vi "Module_ENG_TCPClient.vi"(8 "error in (no error)":errorcluster, 9 "Module ID (-1: Do not Address)":i32=-1, 10 "Wait on Module(s) (\"\": none)":string, 11 "Auto Reconnect?":bool) -> (0 "error out":errorcluster)   [LabVIEW 2019, in "Module_ENG_TCPClient.lvclass"]
doc: "created using\nJSMA Module Template - ENGINE Class 0.2.1.12\nRob Humfeld - Jet Engineering\nCopyright (c) 2020, Jet Engineering"
uses:
  Module_ENG_TCPClient.lvclass
  <userlib>/Jet Engineering/JSMA/Libraries/jModule Class/Typedefs/jModule_TimerConfig STYP.ctl
  <userlib>/Jet Engineering/JSMA/Libraries/jModule Class/Typedefs/jModule_TimerType STYP.ctl
  Private/Module_ENG_TCPClient_jMsgTxList STYP.ctl
  <userlib>/Jet Engineering/JSMA/Libraries/jMsg_CORE/jMsg_JSMA_ModuleOnline/jMsg_JSMA_ModuleOnline.lvclass
  Shared/jMsgs/jMsg_TCPConnection_Status/jMsg_TCPConnection_Status.lvclass
  C:/Program Files/National Instruments/LabVIEW 2019/user.lib/Jet Engineering/JSMA/Libraries/jMsg Class/jMsg.lvclass
  Shared/jMsgs/jMsg_TCPClient_Message_Receive/jMsg_TCPClient_Message_Receive.lvclass
  Private/Module_ENG_TCPClient_jMsgRxList STYP.ctl
  <userlib>/Jet Engineering/JSMA/Libraries/jMsg_CORE/jMsg_JSMA_ApplicationShutdown/jMsg_JSMA_ApplicationShutdown.lvclass
  Shared/jMsgs/jMsg_TCPClient_Message_Send/jMsg_TCPClient_Message_Send.lvclass
  Shared/jMsgs/jMsg_TCPClient_Connection_Update/jMsg_TCPClient_Connection_Update.lvclass
  C:/Program Files/National Instruments/LabVIEW 2019/user.lib/Jet Engineering/JSMA/Libraries/jModule Class/jModule.lvclass
  Private/Module_ENG_TCPClient_LocalData STYP.ctl
  Private/Module_ENG_TCPClient_EngineStatus STYP.ctl
  Shared/TCPConnectionSettings STYP.ctl
  Shared/TCPReceiver/TCPReceiver.lvclass
  <userlib>/Jet Engineering/JET_QSM/Code/Private/JET_QSM_InvalidOption STYP.ctl
  <userlib>/Jet Engineering/JSMA/Libraries/jModule Class/jModule.lvclass/jModule.ctl
  Module_ENG_TCPClient.lvclass/Module_ENG_TCPClient.ctl
  Shared/jMsgs/jMsg_TCPClient_Message_Send/jMsg_TCPClient_Message_Send.lvclass/jMsg_TCPClient_Message_Send.ctl
  Shared/jMsgs/jMsg_TCPClient_Connection_Update/jMsg_TCPClient_Connection_Update.lvclass/jMsg_TCPClient_Connection_Update.ctl
  <userlib>/Jet Engineering/JSMA/Libraries/jMsg Class/jMsg.lvclass/jMsg.ctl
  Shared/jMsgs/jMsg_TCPConnection_Status/jMsg_TCPConnection_Status.lvclass/jMsg_TCPConnection_Status.ctl
  <userlib>/Jet Engineering/JSMA/Libraries/jMsg_CORE/jMsg_JSMA_Exception/jMsg_JSMA_Exception.lvclass/jMsg_JSMA_Exception.ctl
  <userlib>/Jet Engineering/JSMA/Libraries/jMsg_CORE/jMsg_JSMA_SubscriptionChange/jMsg_JSMA_SubscriptionChange.lvclass/jMsg_JSMA_SubscriptionChange.ctl
  <userlib>/Jet Engineering/JSMA/Libraries/jMsg_CORE/jMsg_Addressed/jMsg_Addressed.lvclass/jMsg_Addressed.ctl
  Shared/TCPPacket/TCPPacket.lvclass
  Shared/jMsgs/jMsg_TCPClient_Message_Receive/jMsg_TCPClient_Message_Receive.lvclass/jMsg_TCPClient_Message_Receive.ctl
  <userlib>/Jet Engineering/JET_QSM/Code/Private/JET_QSM - Add State [String API].vi
  <userlib>/Jet Engineering/JSMA/Libraries/jModule Class/Read Timeout Configuration.vi
  <userlib>/Jet Engineering/JET_QSM/Code/Private/JET_QSM - Add State to Front [String API].vi
  <userlib>/Jet Engineering/JSMA/Libraries/jModule Class/Read jMsgRx.vi
  <userlib>/Jet Engineering/JSMA/Libraries/jMsg Class/(create) jMsg.vi
  <userlib>/Jet Engineering/JSMA/Libraries/jMsg_CORE/jMsg_JSMA_Exception/(create) jMsg_JSMA_Exception.vi
  <userlib>/Jet Engineering/JSMA/Libraries/jModule Class/jModule - Stats_Exception Count Increment.vi
  <userlib>/Jet Engineering/JSMA/Libraries/jModule Class/jModule - SimpleTx.vi
  <userlib>/Jet Engineering/JSMA/Libraries/jModule Class/jModule - Exception Enqueue.vi
  <userlib>/Jet Engineering/JSMA/Libraries/jMsg Class/Read No Listener Action.vi
  <userlib>/Jet Engineering/JSMA/Libraries/jModule Class/jModule - ExceptionBatchTx.vi
  <userlib>/Jet Engineering/JSMA/Libraries/jModule Class/jModule - Send to List.vi
  <userlib>/Jet Engineering/JSMA/Libraries/jModule Class/jModule - AddressedTx.vi
  <userlib>/Jet Engineering/JSMA/Libraries/jModule Class/jModule - Stats_Tx Count Increment.vi
  <userlib>/Jet Engineering/JSMA/Libraries/jMsg Class/Read Type.vi
  <userlib>/Jet Engineering/JSMA/Libraries/jMsg Class/Write SendID.vi
  <userlib>/Jet Engineering/JSMA/Libraries/jMsg Class/Read Name.vi
  <userlib>/Jet Engineering/JSMA/Libraries/jMasterTable_Subscription/jMasterTable_Subscription - Get Queue Type.vi
  <userlib>/Jet Engineering/JSMA/Libraries/jMsg Class/jMsg - Set Source.vi
  <userlib>/Jet Engineering/JSMA/Libraries/Shared/JSMA_GetClassName.vi
  <userlib>/Jet Engineering/JSMA/Libraries/jMsg Class/Read Sent Time.vi
  <userlib>/Jet Engineering/JSMA/Libraries/jMsg Class/Read Source.vi
  <userlib>/Jet Engineering/JSMA/Libraries/jMasterTable_Subscription/jMasterTable_Subscription - Remove Module.vi
  <userlib>/Jet Engineering/JSMA/Libraries/jMsg Class/Write Source.vi
  <userlib>/Jet Engineering/JSMA/Libraries/jMsg_CORE/jMsg_JSMA_SubscriptionChange/(create) jMsg_JSMA_SubscriptionChange.vi
  <userlib>/Jet Engineering/JSMA/Libraries/jMasterTable_Subscription/jMasterTable_Subscription - Get Sub List.vi
  <userlib>/Jet Engineering/JSMA/Libraries/jMsg_CORE/jMsg_Addressed/Read Qualified Name.vi
  <userlib>/Jet Engineering/JSMA/Libraries/jMsg_CORE/jMsg_Addressed/Read RecvID.vi
  <userlib>/Jet Engineering/JSMA/Libraries/jMasterTable_Subscription/jMasterTable_Subscription - Get-Create Queue.vi
  <userlib>/Jet Engineering/JSMA/Libraries/jMasterTable_Message/jMasterTable_Message - Add jMsg.vi
  <userlib>/Jet Engineering/JSMA/Libraries/jMasterTable_Message/jMasterTable_Message - Get-Create Queue.vi
  <userlib>/Jet Engineering/JSMA/Libraries/jMsg_CORE/jMsg_JSMA_Exception/jMsg_JSMA_Exception.lvclass
  <userlib>/Jet Engineering/JSMA/Libraries/jMsg_CORE/jMsg_JSMA_SubscriptionChange/jMsg_JSMA_SubscriptionChange.lvclass
  <userlib>/Jet Engineering/JSMA/Libraries/jMsg_CORE/jMsg_Addressed/jMsg_Addressed.lvclass
  <vilib>/Utility/error.llb/Trim Whitespace.vi
  <vilib>/Utility/error.llb/Error Cluster From Error Code.vi
  <vilib>/Utility/LVClass/Get LV Class Path.vi
  <userlib>/Jet Engineering/JSMA/Libraries/jSubscription Class/jSubscription.lvclass
  <userlib>/Jet Engineering/JSMA/Libraries/jModule Class/jModule.lvclass
  <userlib>/Jet Engineering/JSMA/Libraries/jMsg Class/jMsg.lvclass
panel:
  out "Timer Configuration":T1 {"Expiration Time" format="%<%.3X>T"}
  out "jModule Name":string
  out "iter":i32
  out "Latency, sec.":dbl
  out "RxTime":timestamp format="%<%H:%M:%S%3u>T"
  out "Last Rx Message":string
  out "Recent states before Error (with tick counts)":string
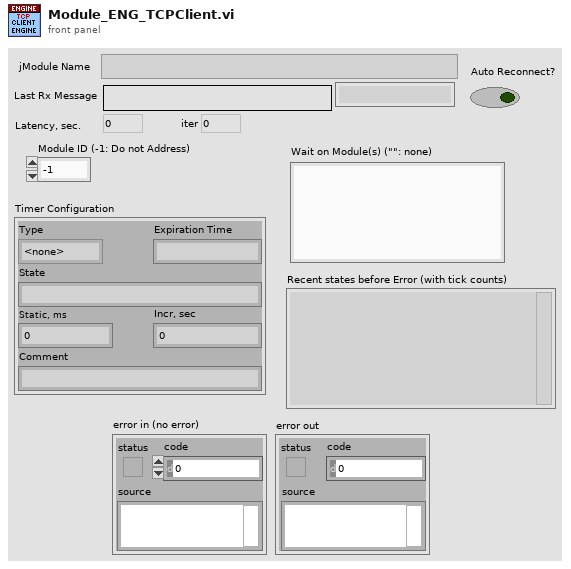
[diagram p1: front panel]
types:
  T1 = typedef "JSMA API.lvlib/jModule.lvclass/jModule_TimerConfig STYP.ctl" = cluster{"Type":T2, "Expiration Time":timestamp, "State":string, "Static, ms":i32, "Incr, sec":dbl, "Comment":string}
  T2 = typedef "JSMA API.lvlib/jModule.lvclass/jModule_TimerType STYP.ctl" = enum16{"<none>", "Static", "Countdown", "Periodic"}
  T3 = typedef "JET_QSM_InvalidOption STYP.ctl" = enum16{"Ignore", "Dialog", "Error"}
  T4 = typedef "Module_ENG_TCPClient.lvclass/Module_ENG_TCPClient_LocalData STYP.ctl" = cluster{"VI":cluster{"error":errorcluster, "isExiting?":bool}, "EngineStatus":T5}
  T5 = typedef "Module_ENG_TCPClient.lvclass/Module_ENG_TCPClient_EngineStatus STYP.ctl" = cluster{"Connection":T6, "Valid Settings?":bool, "Receiver":refnum<class "TCPReceiver.lvclass">}
  T6 = typedef "TCPConnectionSettings STYP.ctl" = cluster{"IP":string, "Port":u16, "Connection":refnum<k5>, "Connected?":bool}
  T7 = typedef "Module_ENG_TCPClient.lvclass/Module_ENG_TCPClient_jMsgRxList STYP.ctl" = cluster{"<placeholder>":refnum<class "jMsg_JSMA_ApplicationShutdown.lvclass">, "jMsg_TCPClient_Message_Send":refnum<class "jMsg_TCPClient_Message_Send.lvclass">, "jMsg_TCPClient_Connection_Update":refnum<class "jMsg_TCPClient_Connection_Update.lvclass">}
  T8 = typedef "Module_ENG_TCPClient.lvclass/Module_ENG_TCPClient_jMsgTxList STYP.ctl" = cluster{"<placeholder>":refnum<class "jMsg_JSMA_ModuleOnline.lvclass">, "jMsg_TCPConnection_Status":refnum<class "jMsg_TCPConnection_Status.lvclass">, "jMsg_TCPClient_Message_Receive":refnum<class "jMsg_TCPClient_Message_Receive.lvclass">}
  T9 = typedef "JET_QSM_Refnum STYP.ctl" = cluster{"state":cluster{"queue":refnum<queue>, "idle":string, "error":string, "STOP":string}, "debug":cluster{"enabled?":bool, "queue":refnum<queue>}, "Invalid.option":T3, "QSM.Name":string}
  T10 = typedef "JET_QSM_Element STYP.ctl" = cluster{"state":string, "data":variant, "comment":string}
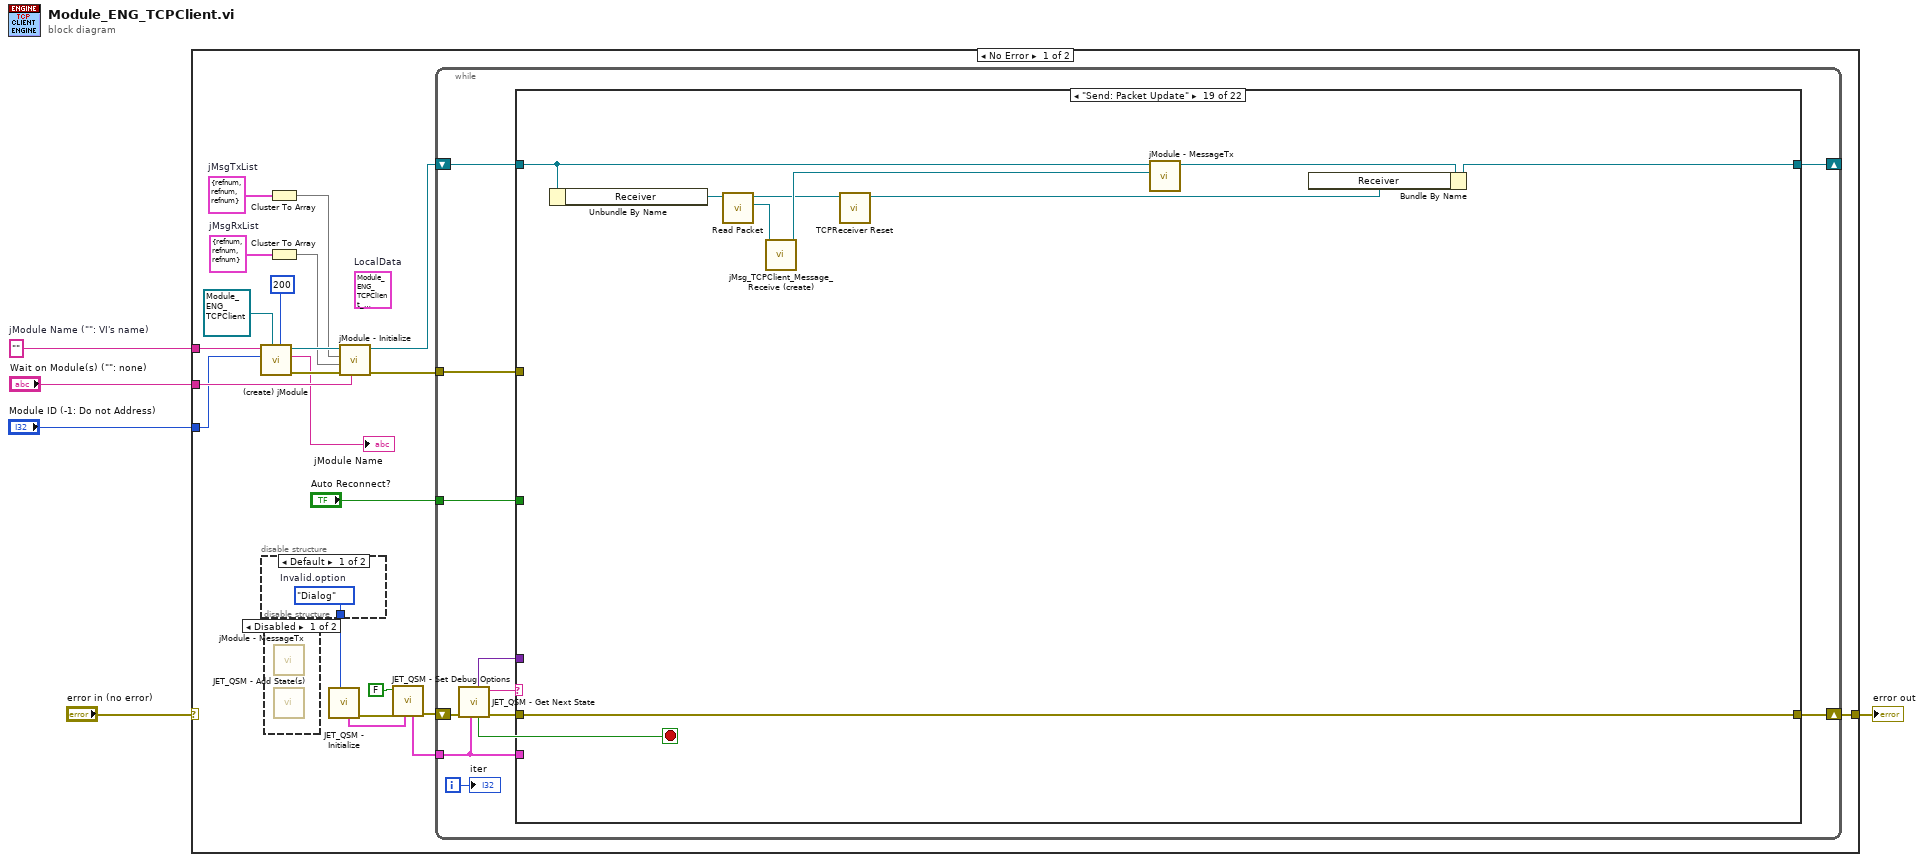
[diagram p0: block diagram]
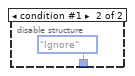
[diagram p3: hidden frame]
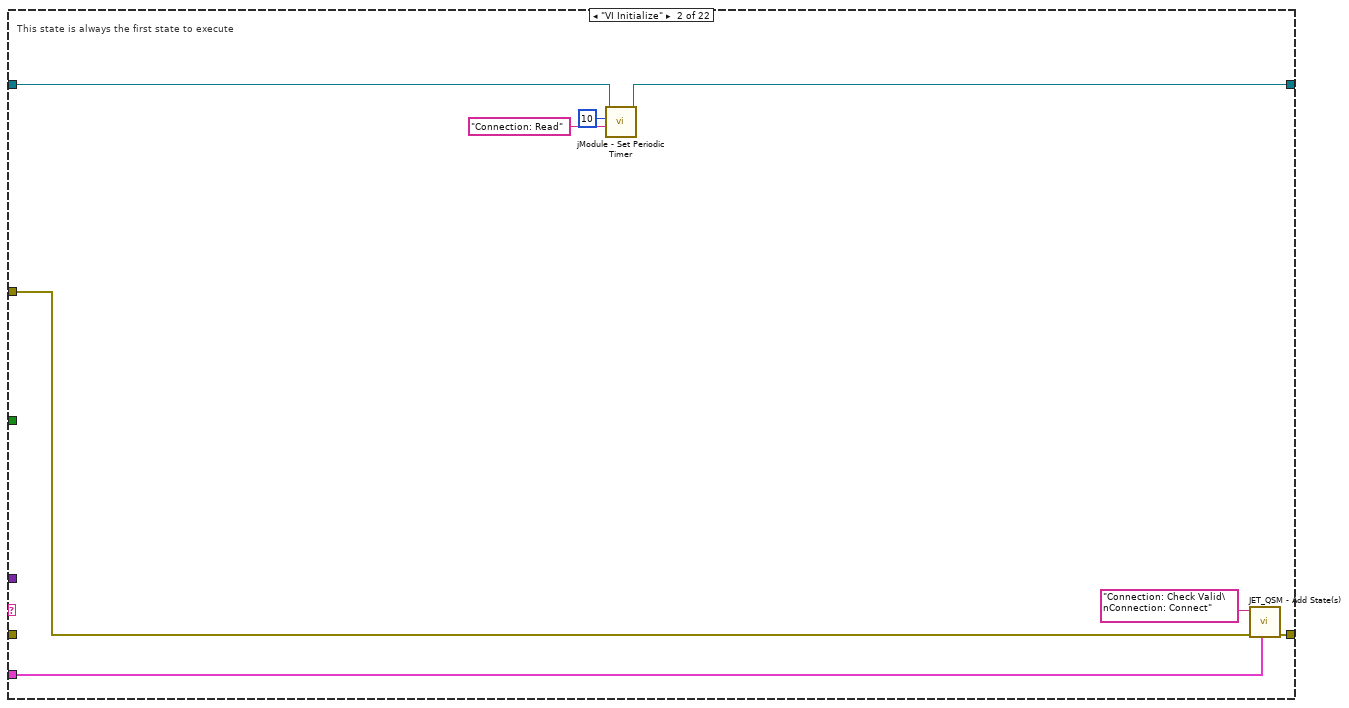
[diagram p5: hidden frame]
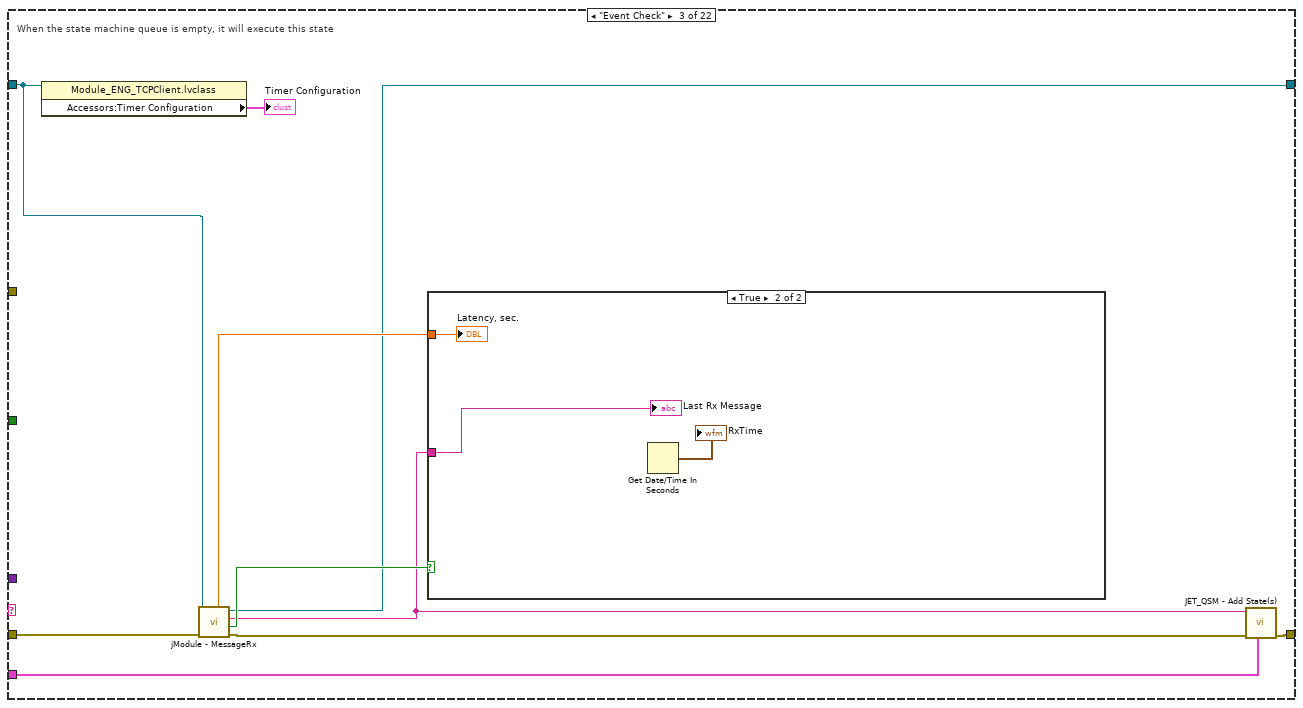
[diagram p6: hidden frame]
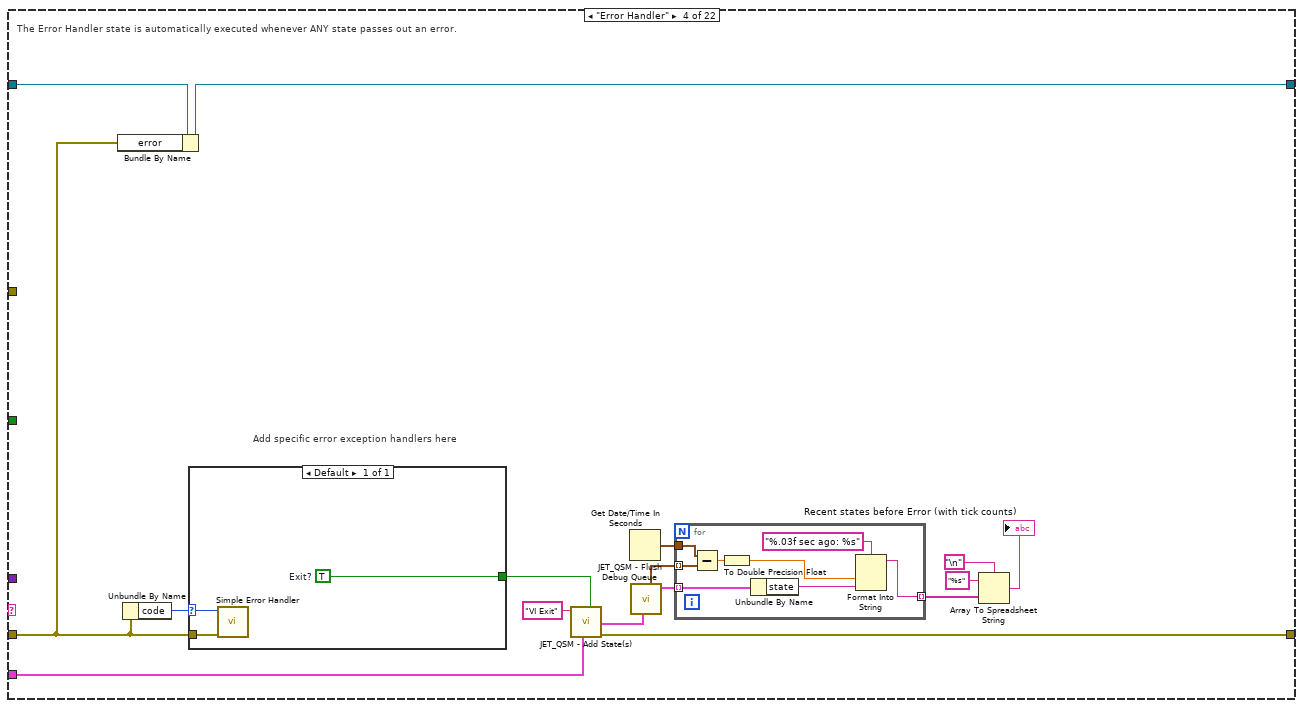
[diagram p8: hidden frame]
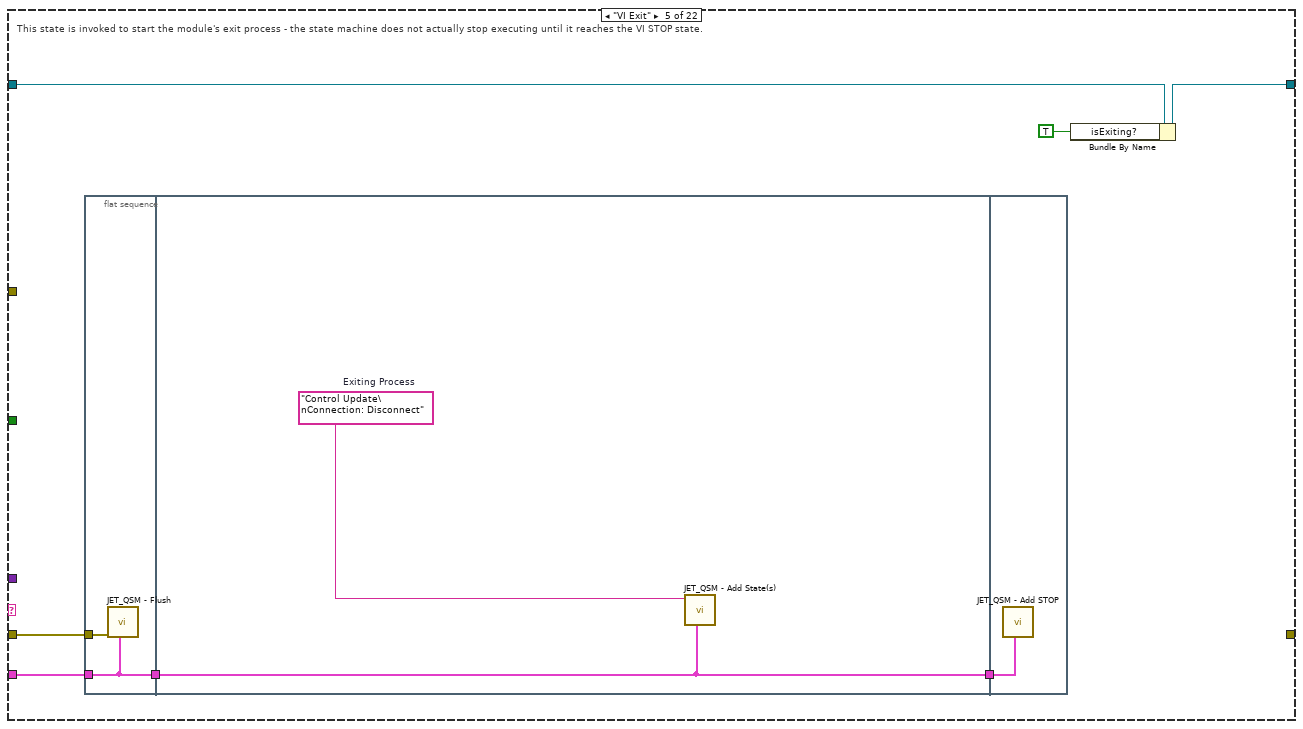
[diagram p9: hidden frame]
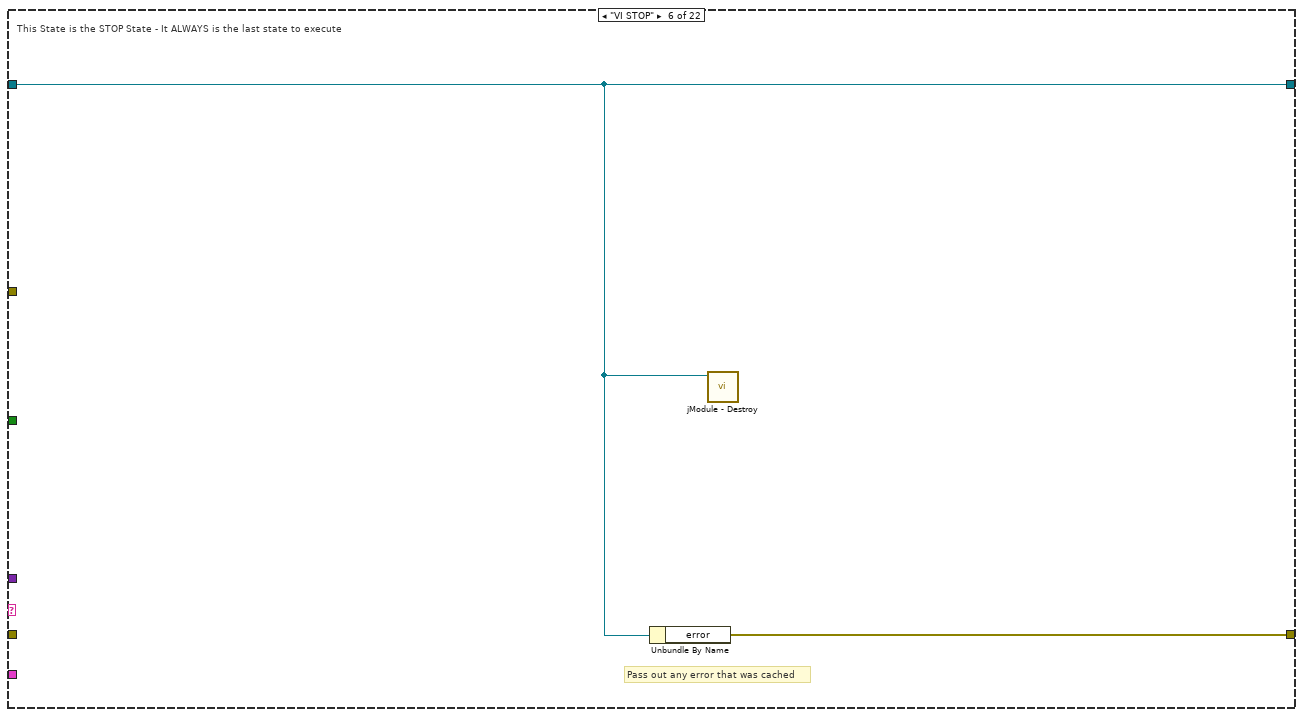
[diagram p10: hidden frame]
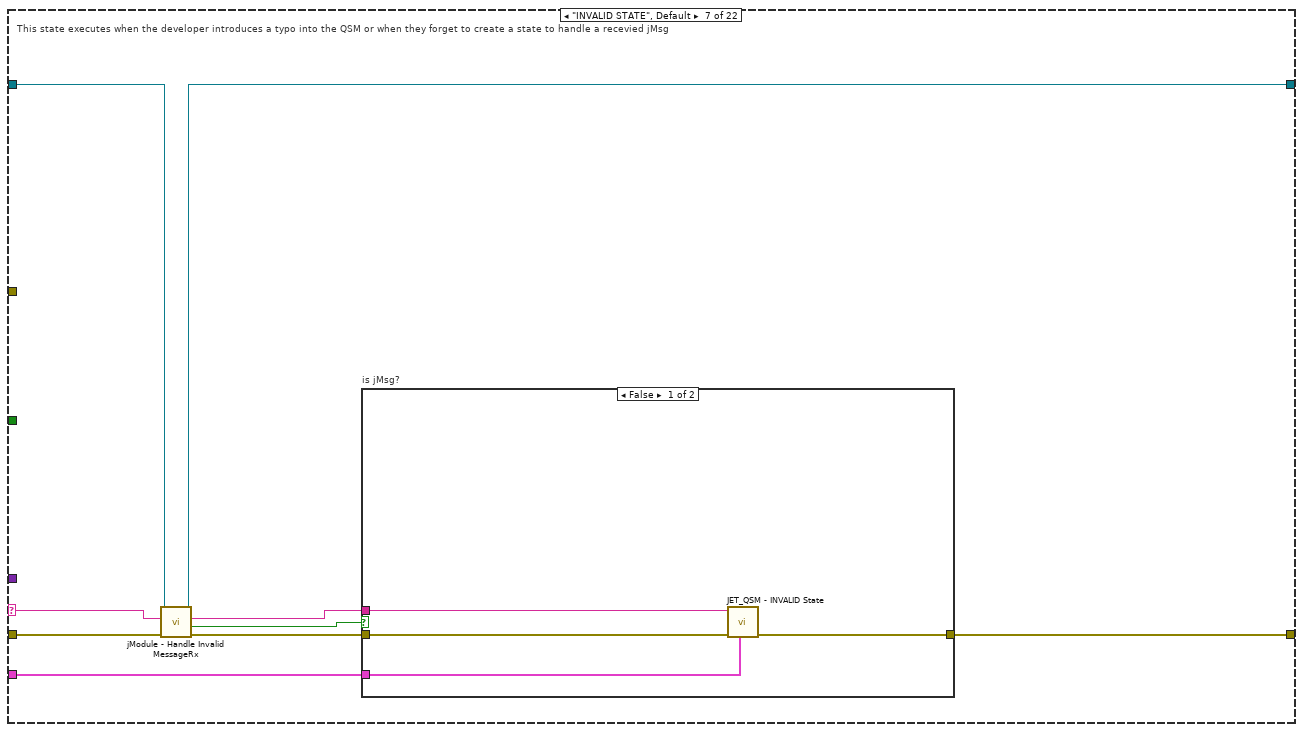
[diagram p11: hidden frame]
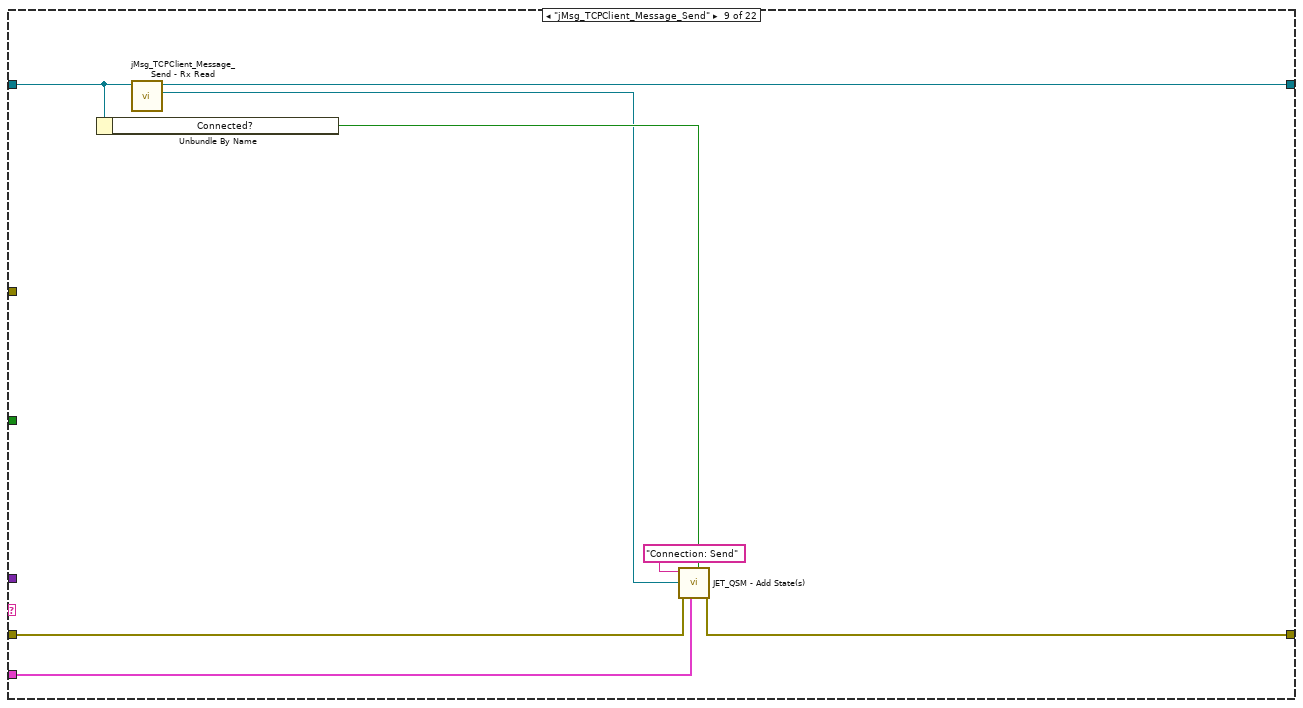
[diagram p14: hidden frame]
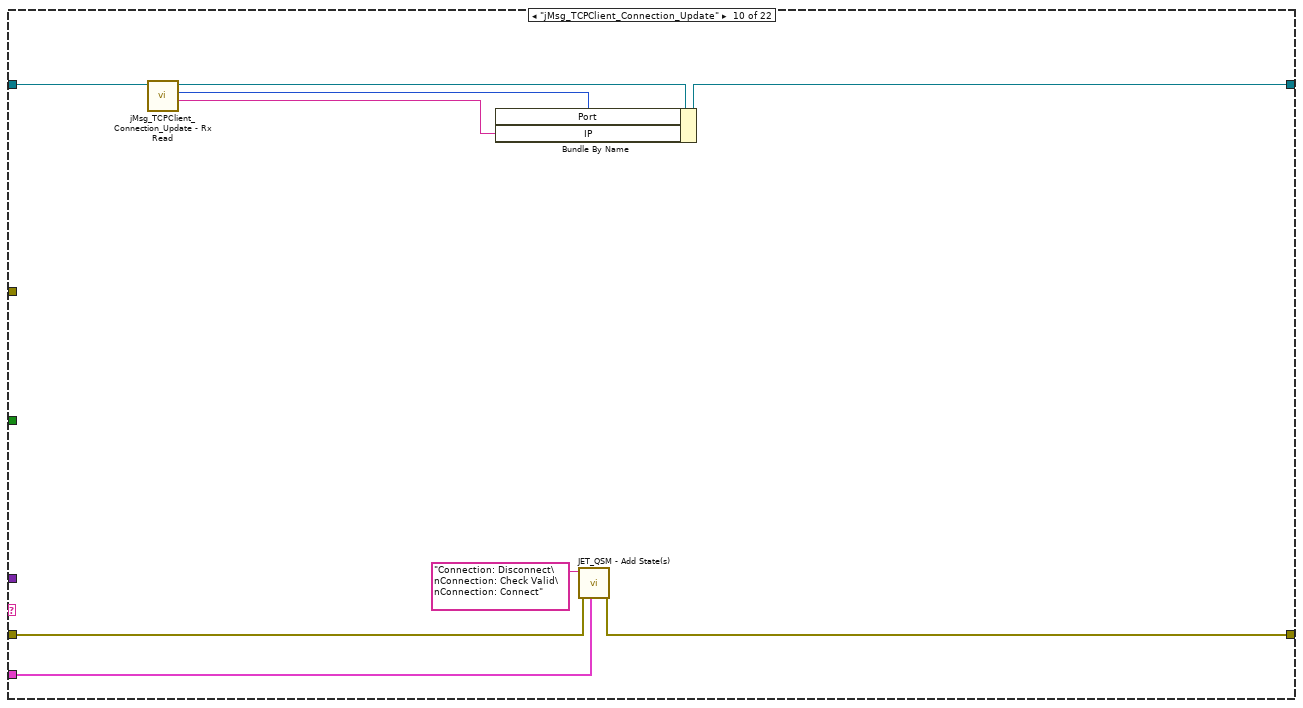
[diagram p15: hidden frame]
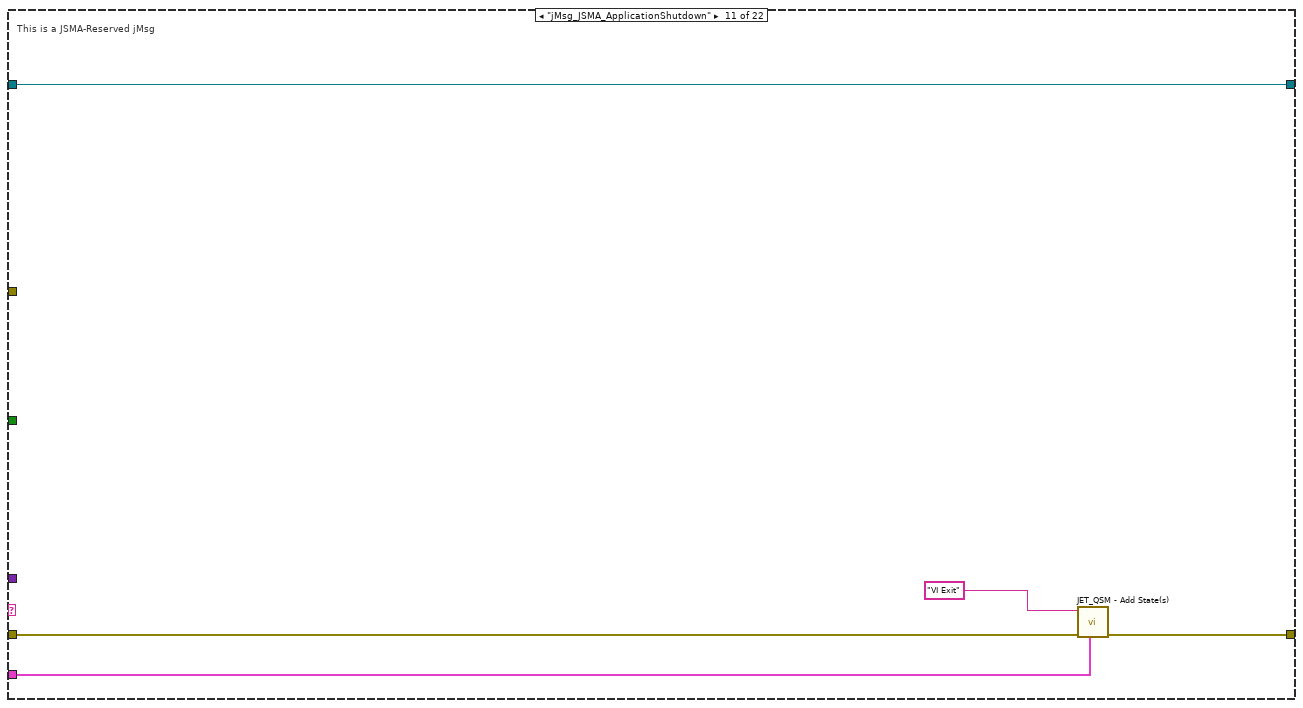
[diagram p16: hidden frame]
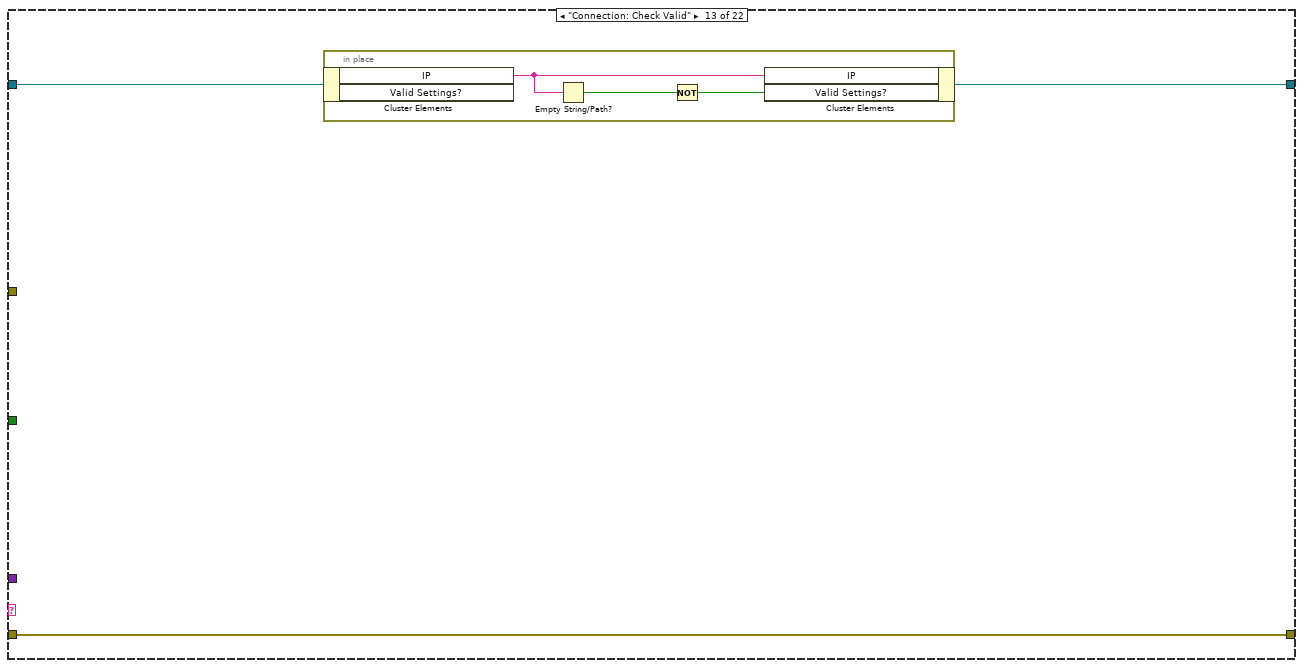
[diagram p18: hidden frame]
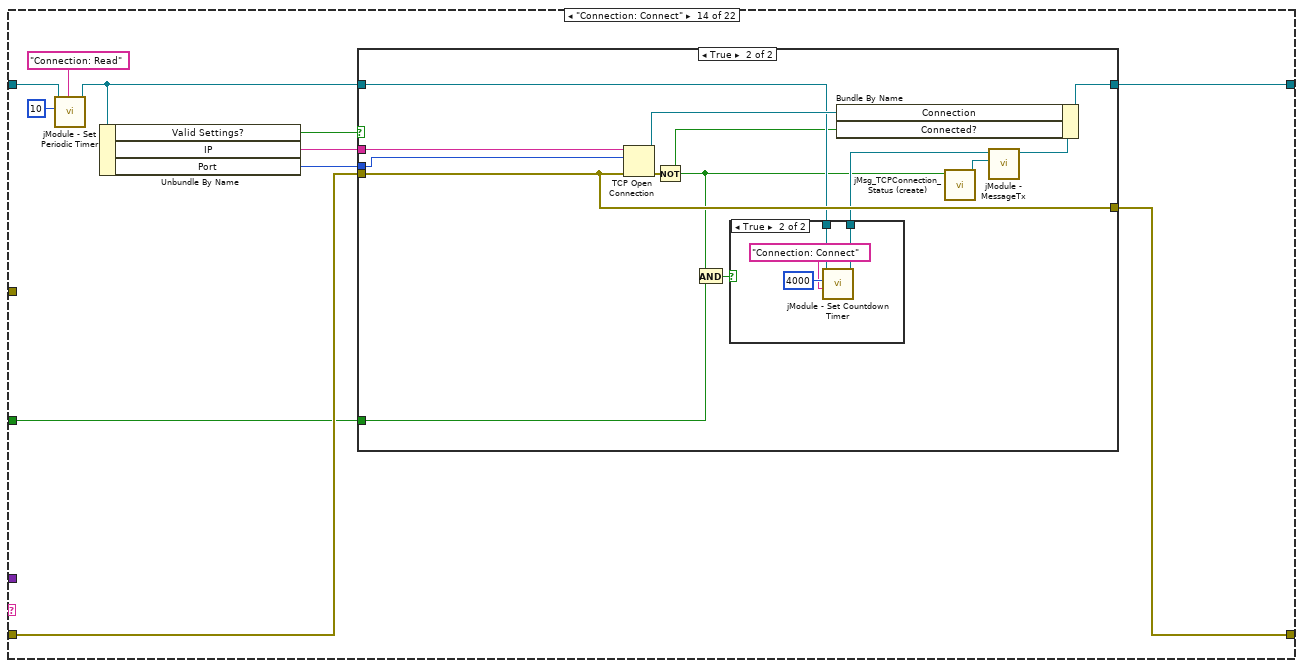
[diagram p19: hidden frame]
diagram:
  w3 = ""  # jModule Name ("": VI's name)
  n1 = case shown="No Error" "error in (no error)" {
    selector: "error in (no error)" -> [_ w268]
    tunnel: [w10 w268] -> w5
    tunnel: "Wait on Module(s) (\"\": none)" -> [w18 _]
    tunnel: w3 -> [w17 _]
    tunnel: "Module ID (-1: Do not Address)" -> [w9 _]
    frame No Error {
      (unwired) T4 {"VI"={"error"={"status"=FALSE, "code"=0, "source"=""}, "isExiting?"=FALSE}, "EngineStatus"={"Connection"={"IP"="", "Port"=0, "Connection"=refnum, "Connected?"=FALSE}, "Valid Settings?"=FALSE, "Receiver"=refnum}}  # LocalData
      w15 = T7 {"<placeholder>"=refnum, "jMsg_TCPClient_Message_Send"=refnum, "jMsg_TCPClient_Connection_Update"=refnum}  # jMsgRxList
      w16 = T8 {"<placeholder>"=refnum, "jMsg_TCPConnection_Status"=refnum, "jMsg_TCPClient_Message_Receive"=refnum}  # jMsgTxList
      n2 = call <userlib>:"(create) jModule.vi"("Max Queue size (50)"=200, "jModule Child class"=refnum<class "Module_ENG_TCPClient.lvclass"> refnum ("jModule Template_ENGINEClass.lvclass"), "Module ID (-1: Do Not Address)"=w9, "jModule Name (\"\": use calling VI's name)"=w17) -> ("error out"=w20:errorcluster, "jModule Name"=→"jModule Name":string, "jModule"=w23:refnum<class "Module_ENG_TCPClient.lvclass">)  [unwired: 4 in, 1 out]
      n3 = disable-structure shown="Default" {
        disable-tunnel: [w28 JET_QSM_InvalidOption_STYP."Ignore" ("Invalid.option (Dialog)")] -> w19
        frame condition #0 (active) {
          w28 = JET_QSM_InvalidOption_STYP."Dialog"  # Invalid.option
        }
        frame condition #1 {
        }
      }
      n4 = disable-structure shown="Disabled" {
        frame Disabled {
          n5 = call <userlib>:"jModule - MessageTx.vi"() -> ()  [unwired: 8 in, 4 out]
          n6 = call-poly <userlib>:"JET_QSM - Add State(s).vi"() -> ()  [unwired: 11 in, 1 out]
        }
        frame Enabled {
        }
      }
      n7 = Cluster To Array(cluster=w16) -> (array=w22:refnum<class "jMsg.lvclass">[])
      n8 = Cluster To Array(cluster=w15) -> (array=w21:refnum<class "jMsg.lvclass">[])
      n9 = call <userlib>:"JET_QSM - Initialize.vi"("invalid state action (Dialog)"=w19) -> ("error out"=w24:errorcluster, "Jet_QSM refnum"=w26:T9)  [unwired: 9 in]
      n10 = call-dynamic "jModule - Initialize.vi"("Wait on Module(s) (\"\": none)"=w18, "error in (no error)"=w20, "jMsgRxList"=w21, "jMsgTxList"=w22, "jModule"=w23) -> ("error out"=w12:errorcluster, "jModule"=w11:refnum<class "Module_ENG_TCPClient.lvclass">)  [unwired: 5 in]
      n11 = call <userlib>:"JET_QSM - Set Debug Options.vi"("Jet_QSM refnum"=w26, "error in (no error)"=w24, "debug.enabled? (F)"=FALSE) -> ("error out"=w13:errorcluster, "Jet_QSM ref"=w25:T9)  [unwired: 7 in]
      n12 = while {
        tunnel: w25 -> [w32]
        shift-right: [w36] -> _
        shift-left: w11 -> [w37]
        shift-right: [w35] -> w10
        shift-left: w13 -> [w41]
        tunnel: w12 -> [w33]
        tunnel: "Auto Reconnect?" -> [w30]
        i -> [w34]
        stop <- w38 stop-if-true
        n13 = call <userlib>:"JET_QSM - Get Next State.vi"("Jet_QSM refnum"=w32, "error in (no error)"=w41) -> ("error out"=w40:errorcluster, "state"=w39:string, "Stop Loop?"=w38:bool, "state data"=w31:variant)  [unwired: 5 in, 1 out]
        n14 = case shown="\"Send: Packet Update\"" w39 {
          selector: w39 -> [_ _ _ _ _ _ w109 _ _ _ _ _ _ _ _ _ _ _ _ _ _ _]
          tunnel: w40 -> [w42 _ w59 w69 w97 _ w110 w119 w127 w133 w138 w143 w147 w156 w192 w195 w211 w242 w258 w259 w261 w266]
          tunnel: w37 -> [w43 w46 w55 w66 w92 w104 w106 w120 w123 w135 w139 w144 w145 w153 w182 w198 w213 w240 w254 w260 w262 w267]
          tunnel: [w43 w47 w53 w65 w91 w104 w105 w120 w124 w136 w139 w144 w146 w158 w186 w199 w214 w243 w252 w260 w262 w267] -> w36
          tunnel: [w42 w51 w60 w72 _ w103 w108 w119 w128 w134 w141 w143 w147 w157 w189 w196 w212 w241 w258 w259 w264 w266] -> w35
          tunnel: w33 -> [_ w49 _ _ _ _ _ _ _ _ _ _ _ _ _ _ _ _ _ _ _ _]
          tunnel: w32 -> [_ w50 w61 w71 w96 _ w107 _ w126 w132 w142 _ _ _ _ _ w210 _ _ _ w265 _]
          tunnel: w31 -> [_ _ _ _ _ _ _ _ _ _ _ _ _ _ _ w201 _ _ _ _ _ _]
          tunnel: w30 -> [_ _ _ _ _ _ _ _ _ _ _ _ _ w155 _ _ _ _ _ _ _ _]
          frame "------ Standard States ------" {
            # "Standard States are required states for a JET_QSM State Machine\n\nTheir names may be changed; use the Initialize function to specify the new names"
            # "This is a section header; the state is never expected to execute"
          }
          frame "VI Initialize" {
            # "This state is always the first state to execute"
            n15 = call <userlib>:"jModule - Set Periodic Timer.vi"("Go to State Periodically (\"\": no change)"="Connection: Read" ("Go to State Periodically (\"\": no change)"), "Timing Period, ms"=u32 10, "jModule"=w46) -> ("jModule"=w47:refnum<class "Module_ENG_TCPClient.lvclass">)  [unwired: 7 in, 1 out]
            n16 = call-poly <userlib>:"JET_QSM - Add State(s).vi"("Jet_QSM refnum"=w50, "error in (no error)"=w49, "state(s)"="Connection: Check Valid\nConnection: Connect") -> ("error out"=w51:errorcluster)  [unwired: 8 in]
          }
          frame "Event Check" {
            # "When the state machine queue is empty, it will execute this state"
            n17 = property class="Module_ENG_TCPClient.lvclass"(reference=w55) -> ("Accessors:Timer Configuration"=→"Timer Configuration":T1)  [unwired: 1 in, 2 out]
            n18 = call-dynamic "jModule - MessageRx.vi"("error in (no error)"=w59, "jModule"=w55) -> ("error out"=w54:errorcluster, "MsgRx?"=w58:bool, "QSMState"=w56:string, "jModule"=w53:refnum<class "Module_ENG_TCPClient.lvclass">, "Latency, sec."=w57:dbl)  [unwired: 4 in, 1 out]
            n19 = case shown="True" w58 {
              tunnel: w56 -> [_ w63]
              tunnel: w57 -> [_ w64]
              frame False {
              }
              frame True {
                n20 = Get Date/Time In Seconds() -> (seconds since 1Jan1904=→"RxTime":timestamp)
                "Last Rx Message" <- w63
                "Latency, sec." <- w64
              }
            }
            n21 = call-poly <userlib>:"JET_QSM - Add State(s).vi"("Jet_QSM refnum"=w61, "error in (no error)"=w54, "state(s)"=w56) -> ("error out"=w60:errorcluster)  [unwired: 8 in]
          }
          frame "Error Handler" {
            # "Add specific error exception handlers here"
            # "The Error Handler state is automatically executed whenever ANY state passes out an error."
            n22 = Bundle By Name(cluster=w66, "error"=w69) -> (w65:refnum<class "Module_ENG_TCPClient.lvclass">)
            n23 = Unbundle By Name(w69) -> ("code"=w67:i32)
            n24 = case shown="Default" w67 {
              selector: w67 -> [w81]
              tunnel: [w82] -> w68
              tunnel: w69 -> [w80]
              frame Default {
                w82 = TRUE  # Exit?
                n25 = call <vilib>:"Simple Error Handler.vi"("error code (no error:0)"=w81, "error in (no error)"=w80) -> ()  [unwired: 3 in, 5 out]
              }
            }
            n26 = call-poly <userlib>:"JET_QSM - Add State(s).vi"("act? (T)"=w68, "Jet_QSM refnum"=w71, "state(s)"="VI Exit") -> ("error out"=w72:errorcluster)  [unwired: 8 in]
            n27 = Get Date/Time In Seconds() -> (seconds since 1Jan1904=w75:timestamp)
            n28 = call <userlib>:"JET_QSM - Flush Debug Queue.vi"("Jet_QSM refnum"=w71) -> ("QSM Elements"=w73:T10[], "Timestamps"=w74:timestamp[])  [unwired: 8 in, 1 out]
            n29 = for {
              tunnel: w73 -> [w90] mode=indexing
              tunnel: [w88] -> w77 mode=indexing
              tunnel: w75 -> [w85]
              tunnel: w74 -> [w86] mode=indexing
              n30 = Subtract(x=w85, y=w86) -> (x-y=w84:dbl)
              n31 = To Double Precision Float(number=w84) -> (double precision float=w83:dbl)
              n32 = Unbundle By Name(w90) -> ("state"=w89:string)
              n33 = Format Into String(format string="%.03f sec ago: %s", w83, w89) -> (resulting string=w88:string)  [unwired: 2 in, 1 out]
            }
            n34 = Array To Spreadsheet String(delimiter (Tab)="\n", array=w77, 3:"%s" ("format string")) -> (spreadsheet string=→"Recent states before Error (with tick counts)":string)
          }
          frame "VI Exit" {
            # "This state is invoked to start the module's exit process - the state machine does not actually stop executing until it reaches the VI STOP state."
            n35 = flat-sequence {
              tunnel: w97 -> [w99]
              tunnel: w96 -> [w98]
              tunnel: [w98] -> w95
              tunnel: w95 -> [w101]
              tunnel: [w101] -> w94
              tunnel: w94 -> [w102]
              frame #0 {
                n36 = call <userlib>:"JET_QSM - Flush.vi"("Jet_QSM ref"=w98, "error in (no error)"=w99) -> ()  [unwired: 8 in, 2 out]
              }
              frame #1 {
                w100 = "Control Update\nConnection: Disconnect"  # Exiting Process
                n37 = call-poly <userlib>:"JET_QSM - Add State(s).vi"("Jet_QSM refnum"=w101, "state(s)"=w100) -> ()  [unwired: 9 in, 1 out]
              }
              frame #2 {
                n38 = call <userlib>:"JET_QSM - Add STOP.vi"("Jet_QSM refnum"=w102) -> ()  [unwired: 10 in, 1 out]
              }
            }
            n39 = Bundle By Name(cluster=w92, "isExiting?"=TRUE ("VI.isExiting?")) -> (w91:refnum<class "Module_ENG_TCPClient.lvclass">)
          }
          frame "VI STOP" {
            # "Pass out any error that was cached"
            # "This State is the STOP State - It ALWAYS is the last state to execute"
            n40 = Unbundle By Name(w104) -> ("error"=w103:errorcluster)
            n41 = call-dynamic "jModule - Destroy.vi"("jModule"=w104) -> ()  [unwired: 10 in, 1 out]
          }
          frame "INVALID STATE", Default {
            # "This state executes when the developer introduces a typo into the QSM or when they forget to create a state to handle a recevied jMsg"
            n42 = call-dynamic "jModule - Handle Invalid MessageRx.vi"("error in (no error)"=w110, "Invalid State"=w109, "jModule"=w106) -> ("error out"=w113:errorcluster, "is jMsg State?"=w111:bool, "Invalid State"=w112:string, "jModule"=w105:refnum<class "Module_ENG_TCPClient.lvclass">)  [unwired: 5 in]
            n43 = case "is jMsg?" shown="False" w111 {
              tunnel: w107 -> [w115 _]
              tunnel: [w114 w118] -> w108
              tunnel: w113 -> [w116 w118]
              tunnel: w112 -> [w117 _]
              frame False {
                n44 = call <userlib>:"JET_QSM - INVALID State.vi"("Jet_QSM refnum"=w115, "error in (no error)"=w116, "state"=w117) -> ("error out"=w114:errorcluster)  [unwired: 8 in]
              }
              frame True {
              }
            }
          }
          frame "------ jMsg  ------" {
            # "This is a section header; the state is never expected to execute"
          }
          frame "jMsg_TCPClient_Message_Send" {
            n45 = Unbundle By Name(w123) -> ("Connected?"=w122:bool)
            n46 = call "jMsg_TCPClient_Message_Send - Rx Read.vi"("jModule"=w123) -> ("Packet"=w121:refnum<class "TCPPacket.lvclass">, "jModule"=w124:refnum<class "Module_ENG_TCPClient.lvclass">)  [unwired: 7 in, 2 out]
            n47 = call-poly <userlib>:"JET_QSM - Add State(s).vi"("act? (T)"=w122, "Jet_QSM refnum"=w126, "error in (no error)"=w127, "state(s) data [ALL states]"=w121, "state(s)"="Connection: Send") -> ("error out"=w128:errorcluster)  [unwired: 6 in]
          }
          frame "jMsg_TCPClient_Connection_Update" {
            n48 = call "jMsg_TCPClient_Connection_Update - Rx Read.vi"("jModule"=w135) -> ("IP Address"=w129:string, "Port"=w130:u16, "jModule"=w137:refnum<class "Module_ENG_TCPClient.lvclass">)  [unwired: 6 in, 2 out]
            n49 = Bundle By Name(cluster=w137, "Port"=w130, "IP"=w129) -> (w136:refnum<class "Module_ENG_TCPClient.lvclass">)
            n50 = call-poly <userlib>:"JET_QSM - Add State(s).vi"("Jet_QSM refnum"=w132, "error in (no error)"=w133, "state(s)"="Connection: Disconnect\nConnection: Check Valid\nConnection: Connect") -> ("error out"=w134:errorcluster)  [unwired: 8 in]
          }
          frame "jMsg_JSMA_ApplicationShutdown" {
            # "This is a JSMA-Reserved jMsg"
            n51 = call-poly <userlib>:"JET_QSM - Add State(s).vi"("Jet_QSM refnum"=w142, "error in (no error)"=w138, "state(s)"="VI Exit") -> ("error out"=w141:errorcluster)  [unwired: 8 in]
          }
          frame "------ Actions  ------" {
            # "This is a section header; the state is never expected to execute"
          }
          frame "Connection: Check Valid" {
            n52 = in-place {
              n53 = in-place-cluster #1(w145) -> ("IP"=w148:string)  [unwired: 1 out]
              n54 = Empty String/Path?(string/path=w148) -> (empty?=w150:bool)
              n55 = Not(x=w150) -> (.not. x?=w149:bool)
              n56 = in-place-cluster #1("IP"=w148, "Valid Settings?"=w149) -> (w146:refnum<class "Module_ENG_TCPClient.lvclass">)
            }
          }
          frame "Connection: Connect" {
            n57 = call <userlib>:"jModule - Set Periodic Timer.vi"("Go to State Periodically (\"\": no change)"="Connection: Read" ("Go to State Periodically (\"\": no change)"), "Timing Period, ms"=u32 10, "jModule"=w153) -> ("jModule"=w154:refnum<class "Module_ENG_TCPClient.lvclass">)  [unwired: 7 in, 1 out]
            n58 = Unbundle By Name(w154) -> ("Valid Settings?"=w161:bool, "IP"=w160:string, "Port"=w159:u16)
            n59 = case shown="True" w161 {
              tunnel: w160 -> [_ w174]
              tunnel: w159 -> [_ w173]
              tunnel: w154 -> [w163 w170]
              tunnel: [w163 w176] -> w158
              tunnel: w156 -> [w162 w171]
              tunnel: [w162 w171] -> w157
              tunnel: w155 -> [_ w168]
              frame False {
              }
              frame True {
                n60 = TCP Open Connection(address=w174, remote port or service name=w173, error in (no error)=w171) -> (connection ID=w175:refnum<k5>, error out=w172:errorcluster)  [unwired: 2 in]
                n61 = Not(x=w172) -> (.not. x?=w164:bool)
                n62 = And(x=w164, y=w168) -> (x .and. y?=w169:bool)
                n63 = case shown="True" w169 {
                  tunnel: [w177 w181] -> w167
                  tunnel: w170 -> [w177 w180]
                  frame False {
                  }
                  frame True {
                    n64 = call <userlib>:"jModule - Set Countdown Timer.vi"("Go to State after Timeout"="Connection: Connect", "Timeout, ms"=u32 4000, "jModule"=w180) -> ("jModule"=w181:refnum<class "Module_ENG_TCPClient.lvclass">)  [unwired: 6 in, 2 out]
                  }
                }
                n65 = call "jMsg_TCPConnection_Status (create).vi"("Connected?"=w164) -> ("jMsg_TCPConnection_Status"=w165:refnum<class "jMsg_TCPConnection_Status.lvclass">)  [unwired: 9 in, 1 out]
                n66 = call <userlib>:"jModule - MessageTx.vi"("jMsg"=w165, "jModule"=w167) -> ("jModule"=w166:refnum<class "Module_ENG_TCPClient.lvclass">)  [unwired: 6 in, 3 out]
                n67 = Bundle By Name(cluster=w166, "Connection"=w175, "Connected?"=w164) -> (w176:refnum<class "Module_ENG_TCPClient.lvclass">)
              }
            }
          }
          frame "Connection: Disconnect" {
            w185 = FALSE ("My.EngineStatus.Connection.Connected?")
            n68 = Unbundle By Name(w182) -> ("Connection"=w190:refnum<k5>, "Connected?"=w191:bool)
            n69 = case shown="True" w191 {
              tunnel: w190 -> [_ w194]
              tunnel: [_ w193] -> w188
              frame False {
              }
              frame True {
                n70 = TCP Close Connection(connection ID=w194) -> (error out=w193:errorcluster)  [unwired: 2 in, 1 out]
              }
            }
            n71 = call <userlib>:"jModule - Set Static Timer.vi"("jModule"=w182) -> ("jModule"=w183:refnum<class "Module_ENG_TCPClient.lvclass">)  [unwired: 9 in, 1 out]
            n72 = Bundle By Name(cluster=w183, "Connected?"=w185) -> (w187:refnum<class "Module_ENG_TCPClient.lvclass">)
            n73 = Merge Errors(w188, w192) -> (w189:errorcluster)
            n74 = call "jMsg_TCPConnection_Status (create).vi"("Connected?"=w185) -> ("jMsg_TCPConnection_Status"=w184:refnum<class "jMsg_TCPConnection_Status.lvclass">)  [unwired: 9 in, 1 out]
            n75 = call <userlib>:"jModule - MessageTx.vi"("jMsg"=w184, "jModule"=w187) -> ("jModule"=w186:refnum<class "Module_ENG_TCPClient.lvclass">)  [unwired: 6 in, 3 out]
          }
          frame "Connection: Send" {
            n76 = Variant To Data(type=refnum<class "TCPPacket.lvclass"> refnum ("TCPPacket.lvclass"), Variant=w201) -> (data=w197:refnum<class "TCPPacket.lvclass">)  [unwired: 1 in, 1 out]
            n77 = in-place {
              in-place-border: w197 -> [w207]
              in-place-border: w195 -> [w203]
              in-place-border: [w202] -> w196
              n78 = in-place-cluster #2(w198) -> ("Connection"=w209:refnum<k5>)
              n79 = call-dynamic "TCPPacket Encode.vi"("error in (no error)"=w203, "TCPPacket in"=w207) -> ("error out"=w204:errorcluster, "Data"=w206:u8[])  [unwired: 7 in, 1 out]
              n80 = Byte Array To String(unsigned byte array=w206) -> (string=w205:string)
              n81 = TCP Write(connection ID=w209, data in=w205, error in (no error)=w204) -> (connection ID out=w208:refnum<k5>, error out=w202:errorcluster)  [unwired: 1 in, 1 out]
              n82 = in-place-cluster #2("Connection"=w208) -> (w199:refnum<class "Module_ENG_TCPClient.lvclass">)
            }
          }
          frame "Connection: Read" {
            n83 = in-place {
              in-place-border: w211 -> [w219]
              in-place-border: [w218] -> w212
              in-place-border: w210 -> [w217]
              n84 = in-place-cluster #3(w213) -> ("Connection"=w222:refnum<k5>, "Receiver"=w220:refnum<class "TCPReceiver.lvclass">, "Connected?"=w215:bool)
              n85 = case shown="True" w215 {
                tunnel: w222 -> [w225 w239]
                tunnel: [w225 w238] -> w221
                tunnel: w220 -> [w224 w234]
                tunnel: w219 -> [w223 w232]
                tunnel: [w223 w231] -> w218
                tunnel: w217 -> [_ w230]
                tunnel: [w224 w227] -> w216
                frame False {
                }
                frame True {
                  n86 = TCP Read(connection ID=w239, bytes to read=1024, error in (no error)=w232, 9:1 ("timeout ms (25000)")) -> (connection ID out=w238:refnum<k5>, data out=w235:string)  [unwired: 1 in, 1 out]
                  n87 = String To Byte Array(string=w235) -> (unsigned byte array=w233:u8[])
                  n88 = call-dynamic "TCPReceiver Receive Bytes.vi"("Data"=w233, "TCPReceiver in"=w234) -> ("TCPReceiver out"=w228:refnum<class "TCPReceiver.lvclass">)  [unwired: 8 in, 1 out]
                  n89 = call-dynamic "Read Done_.vi"("TCPReceiver in"=w228) -> ("Done?"=w229:bool, "TCPReceiver out"=w227:refnum<class "TCPReceiver.lvclass">)  [unwired: 8 in, 1 out]
                  n90 = call-poly <userlib>:"JET_QSM - Add State(s).vi"("act? (T)"=w229, "Jet_QSM refnum"=w230, "state(s)"="Send: Packet Update") -> ("error out"=w231:errorcluster)  [unwired: 8 in]
                }
              }
              n91 = in-place-cluster #3("Connection"=w221, "Receiver"=w216, "Connected?"=w215) -> (w214:refnum<class "Module_ENG_TCPClient.lvclass">)
            }
          }
          frame "Send: Status Update" {
            # "This is how your engine broadcasts its status to the application"
            n92 = disable-structure shown="Disabled" {
              disable-tunnel: [w246 w249] -> w243
              disable-tunnel: w242 -> [w245 w248]
              disable-tunnel: [w244 w248] -> w241
              disable-tunnel: w240 -> [w247 w249]
              frame Disabled {
                # "Create a jMsg\nfor this"
                n93 = Unbundle By Name(w247) -> ()  [unwired: 1 out]
                n94 = call <userlib>:"jModule - MessageTx.vi"("error in (no error)"=w245, "jModule"=w247) -> ("error out"=w244:errorcluster, "jModule"=w246:refnum<class "Module_ENG_TCPClient.lvclass">)  [unwired: 6 in, 2 out]
              }
              frame Enabled {
              }
            }
          }
          frame "Send: Packet Update" {
            n95 = Unbundle By Name(w254) -> ("Receiver"=w257:refnum<class "TCPReceiver.lvclass">)
            n96 = call-dynamic "Read Packet.vi"("TCPReceiver in"=w257) -> ("TCPPacket.lvclass"=w256:refnum<class "TCPPacket.lvclass">, "TCPReceiver out"=w251:refnum<class "TCPReceiver.lvclass">)  [unwired: 8 in, 1 out]
            n97 = call "jMsg_TCPClient_Message_Receive (create).vi"("Packet"=w256) -> ("jMsg_TCPClient_Message_Receive"=w253:refnum<class "jMsg_TCPClient_Message_Receive.lvclass">)  [unwired: 9 in, 1 out]
            n98 = call-dynamic "TCPReceiver Reset.vi"("TCPReceiver in"=w251) -> ("TCPReceiver out"=w250:refnum<class "TCPReceiver.lvclass">)  [unwired: 9 in, 1 out]
            n99 = call <userlib>:"jModule - MessageTx.vi"("jMsg"=w253, "jModule"=w254) -> ("jModule"=w255:refnum<class "Module_ENG_TCPClient.lvclass">)  [unwired: 6 in, 3 out]
            n100 = Bundle By Name(cluster=w255, "Receiver"=w250) -> (w252:refnum<class "Module_ENG_TCPClient.lvclass">)
          }
          frame "------ Window and Panel Control ------" {
            # "This is a section header; the state is never expected to execute"
          }
          frame "Control Update" {
            # "Update all control properties values from the status cluster in this state - in this way we can separate the View from the Model and Controller, as well as consolidate/reduce locals and property nodes"
            n101 = call-poly <userlib>:"JET_QSM - Add State(s).vi"("Jet_QSM refnum"=w265, "error in (no error)"=w261, "state(s)"="Indicator Update") -> ("error out"=w264:errorcluster)  [unwired: 8 in]
          }
          frame "Indicator Update" {
            # "Update all indicator properties and values from the status cluster in this state - in this way we can separate the View from the Model and Controller, as well as consolidate/reduce property nodes"
          }
        }
        "iter" <- w34
      }
    }
    frame Error {
    }
  }
  "error out" <- w5
